vi "TLCamera Main.vi"() -> ()   [LabVIEW 2015]
uses:
  Status - Main.ctl
  Controls/Color Modes.ctl
  SubVIs/Parameters Get & Set/Get Parameters/Get CameraSensorType.vi
  Controls/Binning.ctl
  C:/code/Host/Installer/Scientific Camera Interfaces/LabVIEW/32_bit/Library_X86/Thorlabs.TSI.TLCameraInterfaces.dll
  code/Host/Installer/Scientific Camera Interfaces/LabVIEW/32_bit/Library_X86/Thorlabs.TSI.TLCameraInterfaces.dll
  Controls/Trigger Modes.ctl
  Controls/Taps.ctl
  SubVIs/Parameters Get & Set/Set Parameters/Set ExposureTime_us.vi
  SubVIs/Parameters Get & Set/Set Parameters/Set BlackLevel.vi
  SubVIs/Parameters Get & Set/Set Parameters/Set Gain.vi
  SubVIs/Parameters Get & Set/Get Parameters/Get ROIAndBin.vi
  SubVIs/Parameters Get & Set/Get Parameters/Get SensorHeight_pixels.vi
  SubVIs/Parameters Get & Set/Get Parameters/Get BinYRange.vi
  SubVIs/Parameters Get & Set/Get Parameters/Get BinXRange.vi
  SubVIs/Parameters Get & Set/Set Parameters/Set FramesPerTrigger_zeroForUnlimited.vi
  SubVIs/Parameters Get & Set/Set Parameters/Set DataRate.vi
  SubVIs/Parameters Get & Set/Set Parameters/Set ROIAndBin.vi
  SubVIs/Parameters Get & Set/Get Parameters/Get BlackLevelRange.vi
  SubVIs/Parameters Get & Set/Get Parameters/Get ExposureTimeRange_us.vi
  SubVIs/Parameters Get & Set/Get Parameters/Get GainRange.vi
  C:/code/Host/Installer/Scientific Camera Interfaces/LabVIEW/32_bit/Library_X86/Thorlabs.TSI.Demosaicker.dll
  code/Host/Installer/Scientific Camera Interfaces/LabVIEW/32_bit/Library_X86/Thorlabs.TSI.Demosaicker.dll
  C:/code/Host/Installer/Scientific Camera Interfaces/LabVIEW/32_bit/Library_X86/Thorlabs.TSI.ColorProcessor.dll
  code/Host/Installer/Scientific Camera Interfaces/LabVIEW/32_bit/Library_X86/Thorlabs.TSI.ColorProcessor.dll
  C:/code/Host/Installer/Scientific Camera Interfaces/LabVIEW/32_bit/Library_X86/Thorlabs.TSI.ColorInterfaces.dll
  code/Host/Installer/Scientific Camera Interfaces/LabVIEW/32_bit/Library_X86/Thorlabs.TSI.ColorInterfaces.dll
  SubVIs/Color/Color Processor References.ctl
  SubVIs/Parameters Get & Set/Get Parameters/Get BitDepth.vi
  Controls/Color Balance.ctl
  SubVIs/Parameters Get & Set/Set Parameters/Set Taps.vi
  SubVIs/Parameters Get & Set/Get Parameters/Get SensorWidth_pixels.vi
  Controls/Region of Interest.ctl
  Controls/Trigger Polarity.ctl
  Controls/Trigger Settings.ctl
  Controls/Data Rate.ctl
panel:
  out "event callback refnum":refnum<k27>
  out "Status":T1
  in  "Exit":bool
  out "Frame Number":u32
  out "Camera Image":picture
  in  "Camera Settings":T11={"Color Balance"={"Red Gain"=1.0, "Green Gain"=1.0, "Blue Gain"=1.0}, "Region of Interest"={"Origin - X"=0, "Origin - Y"=0, "Width"=1392, "Height"=1040}, "Binning"={"Bin - X"=1, "Bin - Y"=1}, "Frame Settings"={"Frames per Trigger\n(zero for unlimited)"=0}, "Data Rate"={"DataRate"=enum."ReadoutSpeed20MHz", "Taps"=enum."SingleTap"}, "Image Type"=enum."Standard RGB", "Trigger Settings"={"Trigger Mode"=enum."Software", "Trigger Polarity"=enum."ActiveHigh"}, "Exposure (ms)"=100.0, "Gain"=0, "Black Level"=48} {"Black Level" max=100; "Gain" max=1023; "Binning"."Bin - Y" min=1 max=16; "Binning"."Bin - X" min=1 max=16; "Color Balance"."Blue Gain" min=0 max=10 step=0.05 scale=0.0..10.0 scale format="%#_3g"; "Color Balance"."Green Gain" min=0 max=10 step=0.05 scale=0.0..10.0 scale format="%#_3g"; "Color Balance"."Red Gain" min=0 max=10 step=0.05 scale=0.0..10.0 scale format="%#_3g"}
  in  "Close Camera":bool
  in  "Open Camera":bool
  in  "Stop Camera":bool
  in  "Start Camera":bool
  in  "Refresh":bool
  in  "Camera Serial Numbers":u16(ring) items=["1234"]
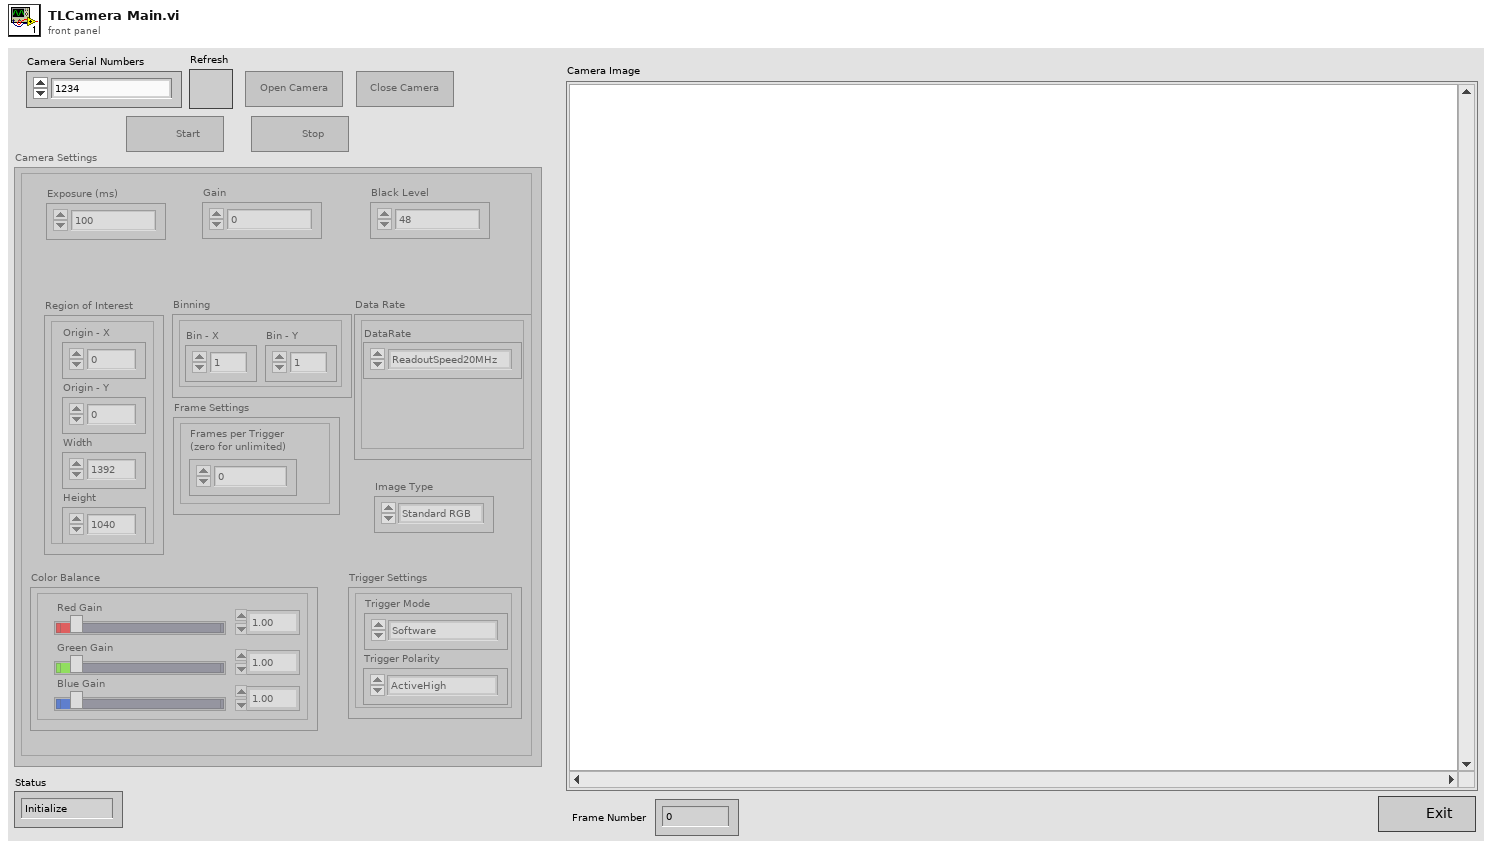
[diagram p1: front panel]
types:
  T1 = typedef "Status - Main.ctl" = enum16{"Initialize", "GUI", "Close"}
  T2 = typedef "Color Balance.ctl" = cluster{"Red Gain":sgl, "Green Gain":sgl, "Blue Gain":sgl}
  T3 = typedef "Region of Interest.ctl" = cluster{"Origin - X":u32, "Origin - Y":u32, "Width":u32, "Height":u32}
  T4 = typedef "Binning.ctl" = cluster{"Bin - X":u32, "Bin - Y":u32}
  T5 = typedef "Data Rate.ctl" = enum32{"ReadoutSpeed20MHz", "ReadoutSpeed40MHz", "FPS30", "FPS50"}
  T6 = typedef "Taps.ctl" = enum32{"SingleTap", "DualTap", "QuadTap"}
  T7 = typedef "Color Modes.ctl" = enum16{"Standard RGB", "Linear RGB", "Unprocessed"}
  T8 = typedef "Trigger Settings.ctl" = cluster{"Trigger Mode":T9, "Trigger Polarity":T10}
  T9 = typedef "Trigger Modes.ctl" = enum16{"Software", "Hardware Standard", "Bulb(PDX) Mode"}
  T10 = typedef "Trigger Polarity.ctl" = enum32{"ActiveHigh", "ActiveLow"}
  T11 = cluster{"Color Balance":T2, "Region of Interest":T3, "Binning":T4, "Frame Settings":cluster{"Frames per Trigger\n(zero for unlimited)":u32}, "Data Rate":cluster{"DataRate":T5, "Taps":T6}, "Image Type":T7, "Trigger Settings":T8, "Exposure (ms)":dbl, "Gain":u32, "Black Level":u32}
  T12 = typedef "Color Processor References.ctl" = cluster{"Demosaicker reference":refnum<k24>, "ColorProcessorSDK reference":refnum<k24>, "StandardRGBColorProcessor":refnum<k24>, "LinearRGBColorProcessor":refnum<k24>}
  T13 = enum8{"Enabled", "Disabled", "Disabled and Grayed Out"}
  T14 = cluster{"TLCamera reference out":refnum<k24>, "Frame Number":refnum<vi>, "Camera Image":refnum<vi>, "Value":T7, "Color Processor References":T12}
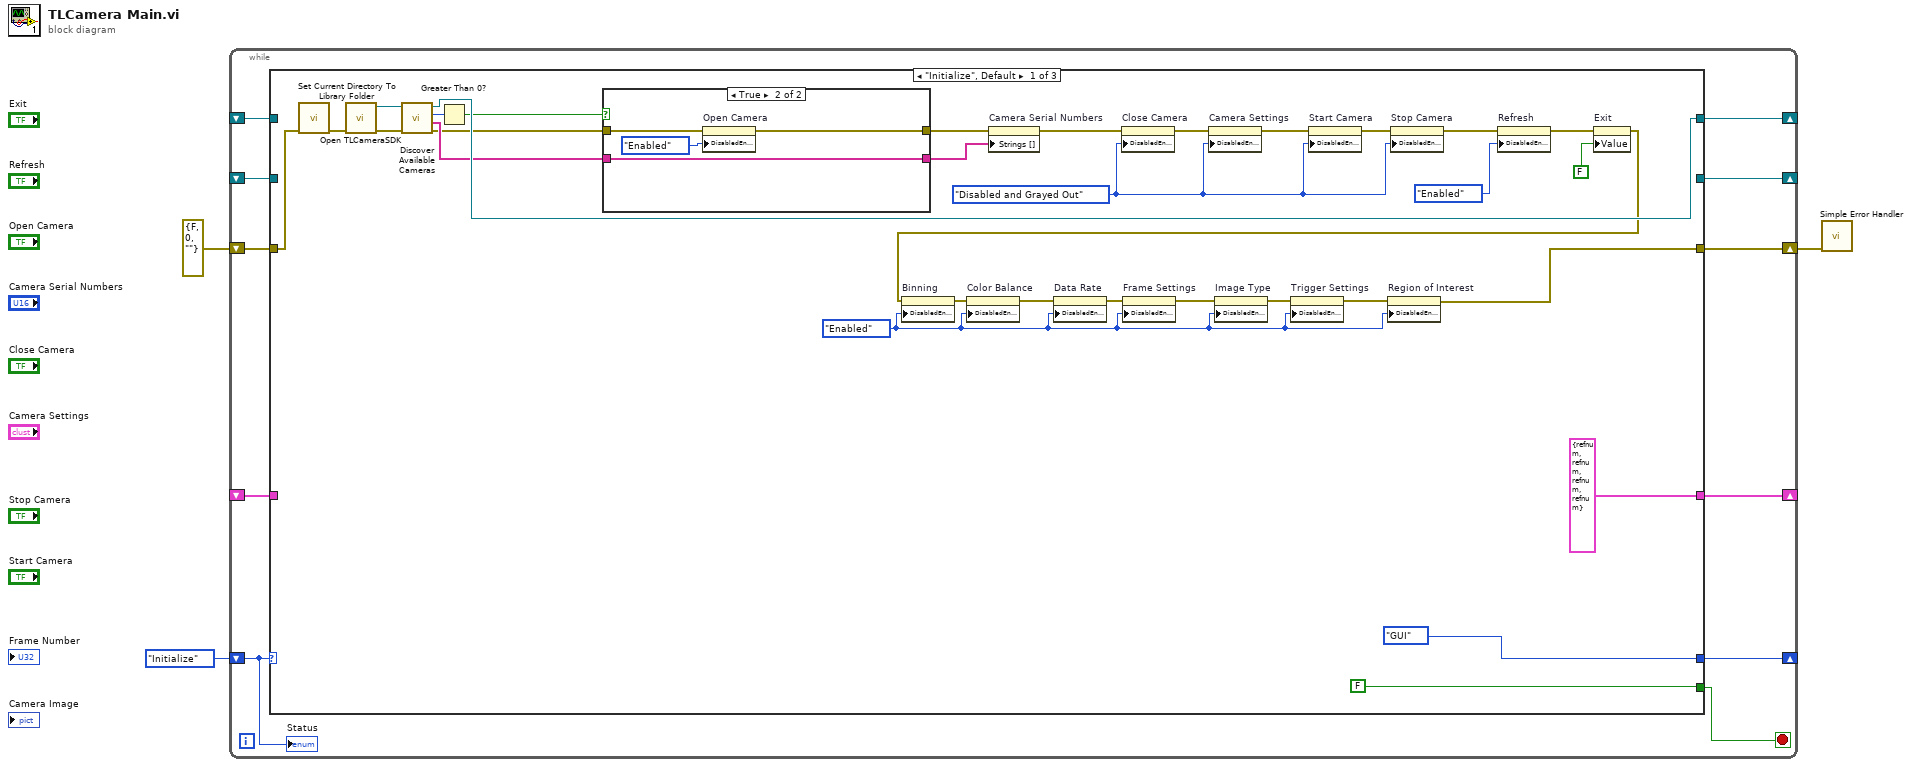
[diagram p0: block diagram]
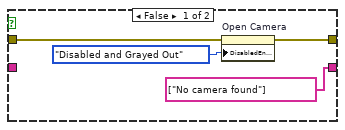
[diagram p2: hidden frame]
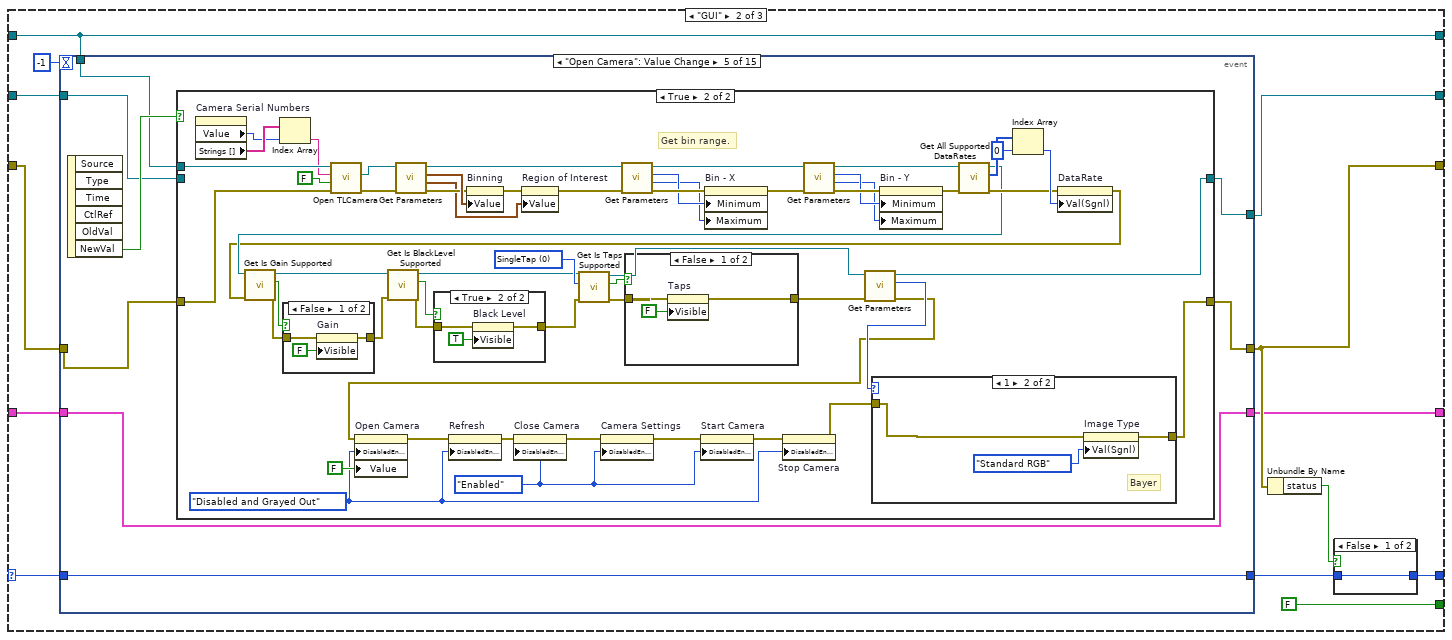
[diagram p3: hidden frame]
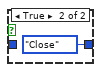
[diagram p4: hidden frame]
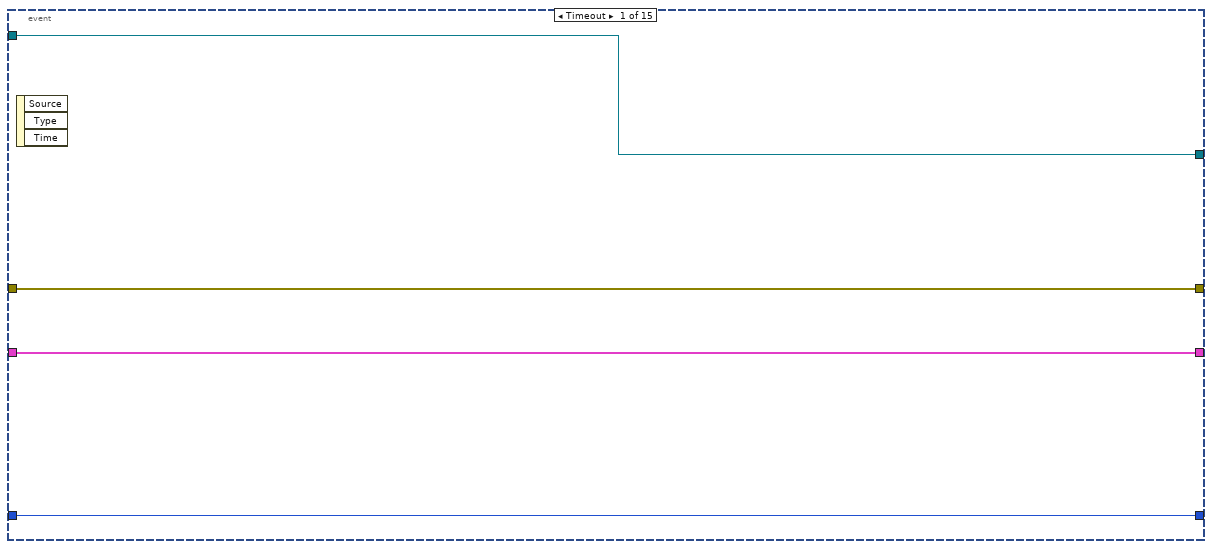
[diagram p5: hidden frame]
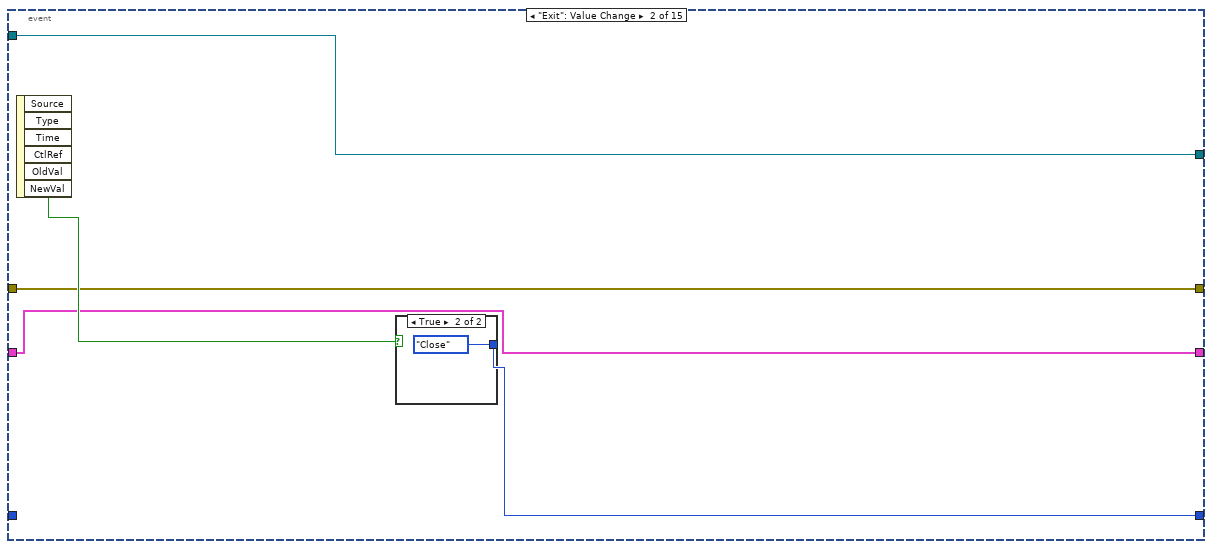
[diagram p6: hidden frame]
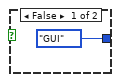
[diagram p7: hidden frame]
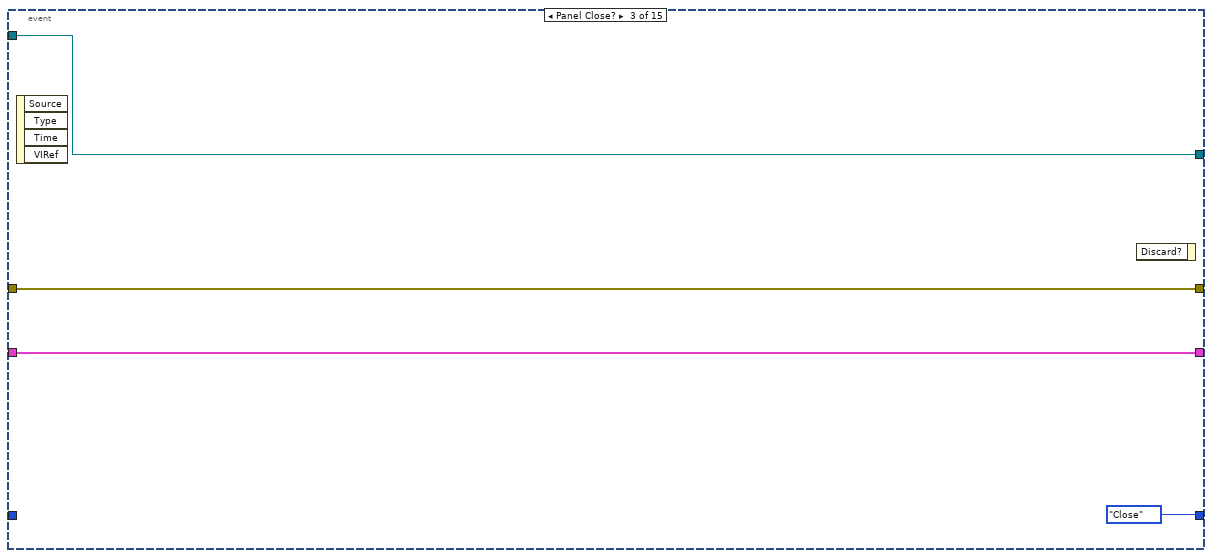
[diagram p8: hidden frame]
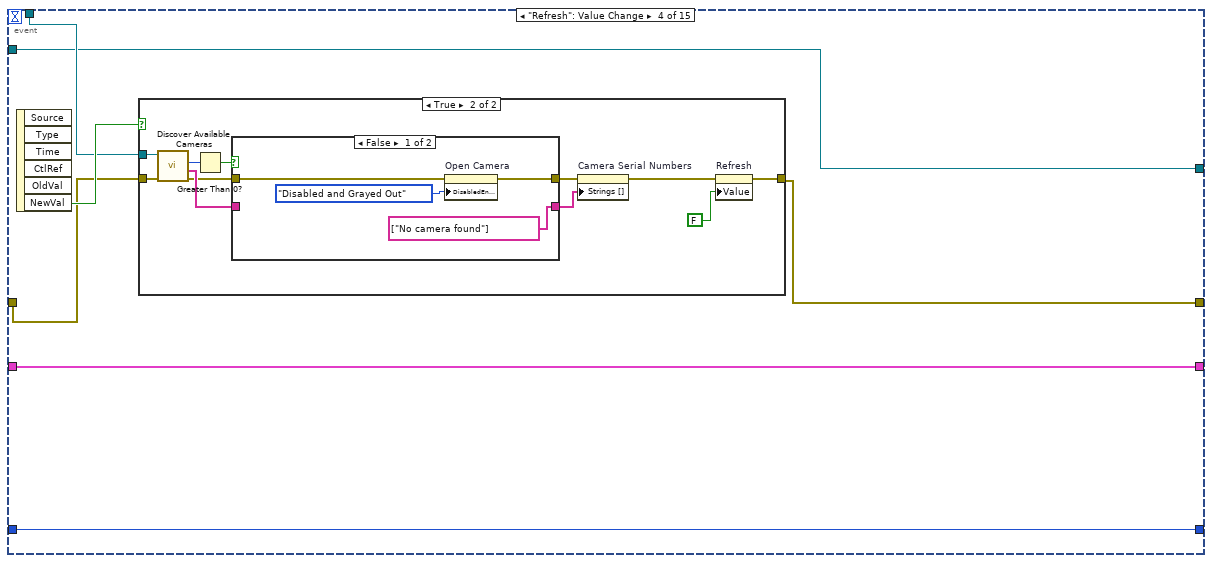
[diagram p9: hidden frame]
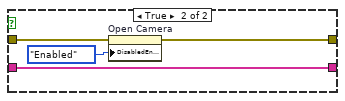
[diagram p11: hidden frame]
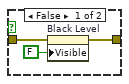
[diagram p13: hidden frame]
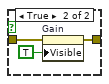
[diagram p14: hidden frame]
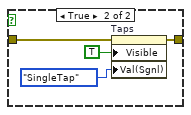
[diagram p15: hidden frame]
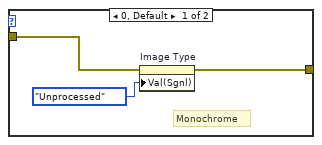
[diagram p16: hidden frame]
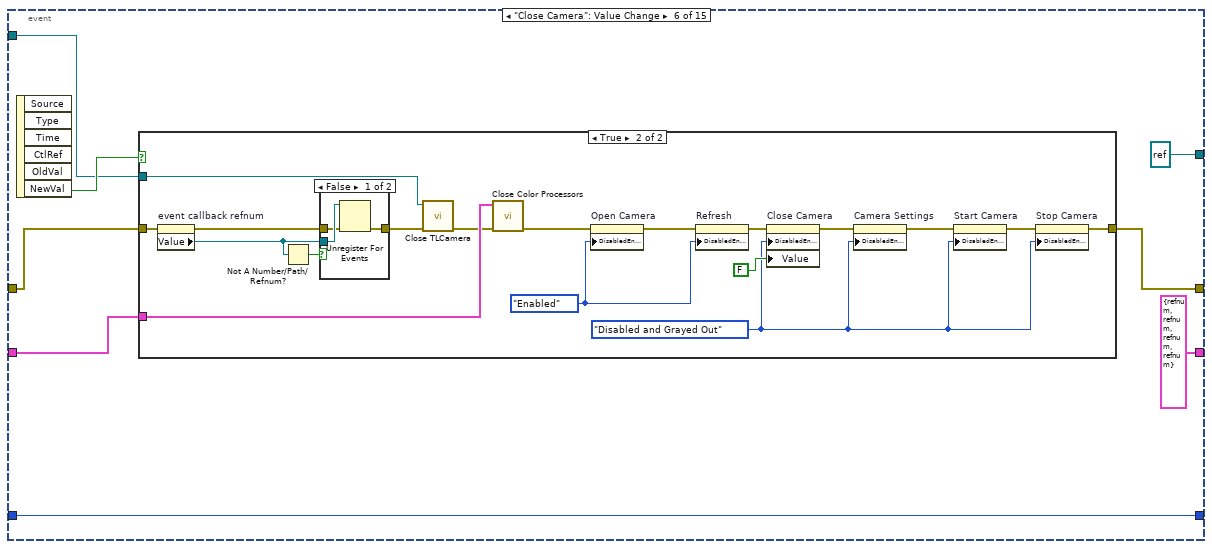
[diagram p17: hidden frame]
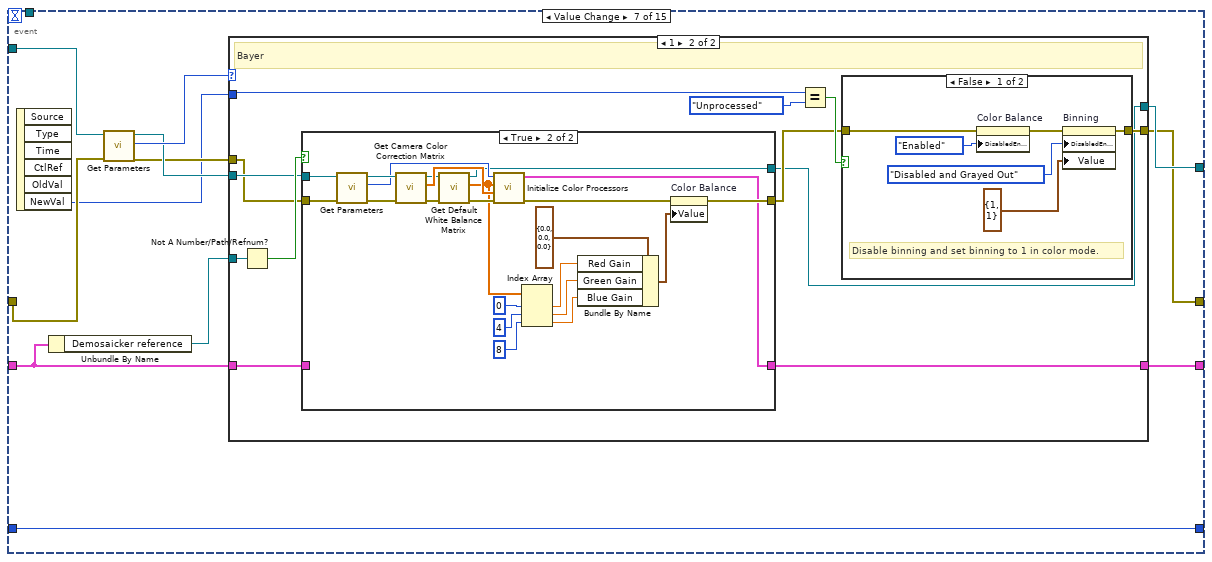
[diagram p20: hidden frame]
diagram:
  n1 = while {
    shift-right: [w7] -> _
    shift-left: Status_-_Main."Initialize" -> [w6]
    shift-right: [w14] -> _
    shift-left: _ -> [w13]
    shift-right: [w11] -> w1
    shift-left: errorcluster {"status"=FALSE, "code"=0, "source"=""} ("error in (no error)") -> [w12]
    shift-right: [w9] -> _
    shift-left: _ -> [w8]
    shift-right: [w4] -> _
    shift-left: _ -> [w5]
    stop <- w10 stop-if-true
    n2 = case shown="\"Initialize\", Default" w6 {
      selector: w6 -> [_ w65 w579]
      tunnel: [w45 w64 _] -> w14
      tunnel: w13 -> [_ w64 w581]
      tunnel: w12 -> [w17 w62 w562]
      tunnel: [w19 w61 w557] -> w11
      tunnel: [FALSE FALSE TRUE] -> w10
      tunnel: [Status_-_Main."GUI" w58 w579] -> w7
      tunnel: [_ w63 _] -> w9
      tunnel: w8 -> [_ w57 w576]
      tunnel: w5 -> [_ w56 w554]
      tunnel: [T12 {"Demosaicker reference"=refnum, "ColorProcessorSDK reference"=refnum, "StandardRGBColorProcessor"=refnum, "LinearRGBColorProcessor"=refnum} ("Color Processor References") w55 T12 {"Demosaicker reference"=refnum, "ColorProcessorSDK reference"=refnum, "StandardRGBColorProcessor"=refnum, "LinearRGBColorProcessor"=refnum} ("Color Processor References")] -> w4
      frame "Initialize", Default {
        w26 = T13."Enabled" ("Disabled")
        w35 = T13."Disabled and Grayed Out" ("Disabled")
        n3 = call "Set Current Directory To Library Folder.vi"("error in (no error)"=w17) -> ("error out"=w18:errorcluster)  [unwired: 10 in]
        n4 = call "Open TLCameraSDK.vi"("error in (no error)"=w18) -> ("error out"=w31:errorcluster, "TLCameraSDK ref out"=w30:refnum<k24>)  [unwired: 9 in]
        n5 = call "Discover Available Cameras.vi"("error in (no error)"=w31, "TLCameraSDK reference"=w30) -> ("error out"=w41:errorcluster, "Serial Numbers"=w43:string[], "Number of Cameras"=w46:i32, "TLCameraSDK reference out"=w45:refnum<k24>)  [unwired: 6 in]
        n6 = Greater Than 0?(x=w46) -> (x > 0?=w44:bool)
        n7 = case shown="True" w44 {
          tunnel: w43 -> [_ w54]
          tunnel: [string[] ["No camera found"] ("Serial Numbers") w54] -> w42
          tunnel: w41 -> [w48 w52]
          tunnel: [w47 w51] -> w40
          frame False {
            n8 = property on="Open Camera" class="Bool (strict)"(error in=w48, "DisabledEnum"=T13."Disabled and Grayed Out" ("Disabled")) -> (error out=w47:errorcluster)  [unwired: 1 in, 1 out]
          }
          frame True {
            n9 = property on="Open Camera" class="Bool (strict)"(error in=w52, "DisabledEnum"=T13."Enabled" ("Disabled")) -> (error out=w51:errorcluster)  [unwired: 1 in, 1 out]
          }
        }
        n10 = property on="Camera Serial Numbers" class="Ring (strict)"(error in=w40, "Strings []"=w42) -> (error out=w39:errorcluster)  [unwired: 1 in, 1 out]
        n11 = property on="Close Camera" class="Bool (strict)"(error in=w39, "DisabledEnum"=w35) -> (error out=w38:errorcluster)  [unwired: 1 in, 1 out]
        n12 = property on="Camera Settings" class="Clust (strict)"(error in=w38, "DisabledEnum"=w35) -> (error out=w37:errorcluster)  [unwired: 1 in, 1 out]
        n13 = property on="Start Camera" class="Bool (strict)"(error in=w37, "DisabledEnum"=w35) -> (error out=w36:errorcluster)  [unwired: 1 in, 1 out]
        n14 = property on="Stop Camera" class="Bool (strict)"(error in=w36, "DisabledEnum"=w35) -> (error out=w29:errorcluster)  [unwired: 1 in, 1 out]
        n15 = property on="Refresh" class="Bool (strict)"(error in=w29, "DisabledEnum"=T13."Enabled" ("Disabled")) -> (error out=w28:errorcluster)  [unwired: 1 in, 1 out]
        n16 = property on="Exit" class="Bool (strict)"(error in=w28, "Value"=FALSE ("Camera Running")) -> (error out=w25:errorcluster)  [unwired: 1 in, 1 out]
        n17 = property on="Binning" class="Clust (strict)"(error in=w25, "DisabledEnum"=w26) -> (error out=w24:errorcluster)  [unwired: 1 in, 1 out]
        n18 = property on="Color Balance" class="Clust (strict)"(error in=w24, "DisabledEnum"=w26) -> (error out=w23:errorcluster)  [unwired: 1 in, 1 out]
        n19 = property on="Data Rate" class="Clust (strict)"(error in=w23, "DisabledEnum"=w26) -> (error out=w16:errorcluster)  [unwired: 1 in, 1 out]
        n20 = property on="Frame Settings" class="Clust (strict)"(error in=w16, "DisabledEnum"=w26) -> (error out=w22:errorcluster)  [unwired: 1 in, 1 out]
        n21 = property on="Image Type" class="Enum (strict)"(error in=w22, "DisabledEnum"=w26) -> (error out=w21:errorcluster)  [unwired: 1 in, 1 out]
        n22 = property on="Trigger Settings" class="Clust (strict)"(error in=w21, "DisabledEnum"=w26) -> (error out=w20:errorcluster)  [unwired: 1 in, 1 out]
        n23 = property on="Region of Interest" class="Clust (strict)"(error in=w20, "DisabledEnum"=w26) -> (error out=w19:errorcluster)  [unwired: 1 in, 1 out]
      }
      frame "GUI" {
        n24 = event shown="[4] \"Open Camera\": Value Change" {
          selector: _ -> [_ _ _ _ _ _ _ _ _ _ _ _ _ _ _]
          dyn-events: _ -> [_ _ _ _ _ _ _ _ _ _ _ _ _ _ _]
          timeout: -1 -> [_ _ _ _ _ _ _ _ _ _ _ _ _ _ _]
          tunnel: [w73 w77 Status_-_Main."Close" w87 w117 w206 w245 w316 w328 w347 w364 w395 w422 w487 w525] -> w59
          tunnel: w65 -> [w73 _ _ w87 w117 w206 w245 w316 w328 w347 w364 w395 w422 w487 w525]
          tunnel: w64 -> [_ _ _ w90 w118 _ _ _ _ _ _ _ _ _ _]
          tunnel: w62 -> [w72 w76 w83 w89 w116 w209 w244 w315 w331 w343 w366 w383 w420 w426 w528]
          tunnel: [w71 w75 w82 w86 w115 refnum<k24> refnum ("TLCamera reference") w239 w307 w319 w336 w356 w378 w423 w474 w527] -> w63
          tunnel: [w72 w76 w83 w88 w114 w208 w238 w308 w318 w335 w357 w379 w424 w471 w526] -> w61
          tunnel: w57 -> [w71 w75 w82 w86 w113 w205 w237 w306 w327 w342 w367 w378 w421 w472 w524]
          tunnel: w56 -> [w70 w74 w81 w85 w112 w203 w234 w304 w317 w333 w355 w377 w418 w437 w522]
          tunnel: [w70 w74 w81 w85 w112 T12 {"Demosaicker reference"=refnum, "ColorProcessorSDK reference"=refnum, "StandardRGBColorProcessor"=refnum, "LinearRGBColorProcessor"=refnum} ("Color Processor References") w235 w304 w317 w333 w355 w377 w418 w437 w522] -> w55
          event Timeout {
            n25 = event-data() -> ()  [unwired: 1 in, 3 out]
          }
          event "Exit": Value Change {
            n26 = event-data() -> ("NewVal"=w78:bool)  [unwired: 1 in, 5 out]
            n27 = case shown="True" w78 {
              tunnel: [Status_-_Main."GUI" Status_-_Main."Close"] -> w77
              frame False {
              }
              frame True {
              }
            }
          }
          event Panel Close? {
            n28 = event-data() -> ()  [unwired: 1 in, 4 out]
            n29 = event-data() -> ()  [unwired: 2 in, 1 out]
          }
          event "Refresh": Value Change {
            n30 = event-data() -> ("NewVal"=w91:bool)  [unwired: 1 in, 5 out]
            n31 = case shown="True" w91 {
              tunnel: w90 -> [_ w103]
              tunnel: w89 -> [w92 w102]
              tunnel: [w92 w93] -> w88
              frame False {
              }
              frame True {
                n32 = call "Discover Available Cameras.vi"("error in (no error)"=w102, "TLCameraSDK reference"=w103) -> ("error out"=w99:errorcluster, "Serial Numbers"=w100:string[], "Number of Cameras"=w101:i32)  [unwired: 6 in, 1 out]
                n33 = Greater Than 0?(x=w101) -> (x > 0?=w96:bool)
                n34 = case shown="False" w96 {
                  tunnel: w100 -> [_ w111]
                  tunnel: [string[] ["No camera found"] ("Serial Numbers") w111] -> w98
                  tunnel: w99 -> [w105 w109]
                  tunnel: [w104 w108] -> w97
                  frame False {
                    n35 = property on="Open Camera" class="Bool (strict)"(error in=w105, "DisabledEnum"=T13."Disabled and Grayed Out" ("Disabled")) -> (error out=w104:errorcluster)  [unwired: 1 in, 1 out]
                  }
                  frame True {
                    n36 = property on="Open Camera" class="Bool (strict)"(error in=w109, "DisabledEnum"=T13."Enabled" ("Disabled")) -> (error out=w108:errorcluster)  [unwired: 1 in, 1 out]
                  }
                }
                n37 = property on="Camera Serial Numbers" class="Ring (strict)"(error in=w97, "Strings []"=w98) -> (error out=w94:errorcluster)  [unwired: 1 in, 1 out]
                n38 = property on="Refresh" class="Bool (strict)"(error in=w94, "Value"=FALSE ("Refresh")) -> (error out=w93:errorcluster)  [unwired: 1 in, 1 out]
              }
            }
          }
          event "Open Camera": Value Change {
            n39 = event-data() -> ("NewVal"=w119:bool)  [unwired: 1 in, 5 out]
            n40 = case shown="True" w119 {
              tunnel: w118 -> [_ w177]
              tunnel: w116 -> [w120 w145]
              tunnel: [w121 w123] -> w115
              tunnel: w113 -> [w121 _]
              tunnel: [w120 w146] -> w114
              frame False {
              }
              frame True {
                w144 = 0 items=["SingleTap", "DualTap", "QuadTap"] ("Taps")
                w164 = T13."Enabled" ("Disabled")
                w165 = T13."Disabled and Grayed Out" ("Disabled")
                # "Get bin range."
                n41 = property on="Camera Serial Numbers" class="Ring (strict)"() -> ("Value"=w175:u16, "Strings []"=w176:string[])  [unwired: 2 in, 2 out]
                n42 = Index Array(array=w176, index=w175) -> (element=w174:string)
                n43 = call "Open TLCamera.vi"("error in (no error)"=w145, "isDiagnosticsMessagesEnabled"=FALSE, "Camera serial number"=w174, "TLCameraSDK reference"=w177) -> ("error out"=w162:errorcluster, "TLCamera reference out"=w161:refnum<k24>)  [unwired: 5 in, 1 out]
                n44 = call-poly "Get Parameters.vi"("error in (no error)"=w162, "TLCamera reference in"=w161) -> ("error out"=w159:errorcluster, "Region of Interest"=w158:T3, "Binning"=w160:T4, "TLCamera reference out"=w147:refnum<k24>)  [unwired: 6 in]
                n45 = property on="Binning" class="Clust (strict)"(error in=w159, "Value"=w160) -> (error out=w157:errorcluster)  [unwired: 1 in, 1 out]
                n46 = property on="Region of Interest" class="Clust (strict)"(error in=w157, "Value"=w158) -> (error out=w148:errorcluster)  [unwired: 1 in, 1 out]
                n47 = call-poly "Get Parameters.vi"("error in (no error)"=w148, "TLCamera reference in"=w147) -> ("error out"=w156:errorcluster, "Maximum"=w154:u32, "Minimum"=w155:u32, "TLCamera reference out"=w152:refnum<k24>)  [unwired: 6 in]
                n48 = property on="Bin - X" class="DigNum (strict)"(error in=w156, "Minimum"=w155, "Maximum"=w154) -> (error out=w153:errorcluster)  [unwired: 1 in, 1 out]
                n49 = call-poly "Get Parameters.vi"("error in (no error)"=w153, "TLCamera reference in"=w152) -> ("error out"=w151:errorcluster, "Maximum"=w149:u32, "Minimum"=w150:u32, "TLCamera reference out"=w143:refnum<k24>)  [unwired: 6 in]
                n50 = property on="Bin - Y" class="DigNum (strict)"(error in=w151, "Minimum"=w150, "Maximum"=w149) -> (error out=w142:errorcluster)  [unwired: 1 in, 1 out]
                n51 = call "Get All Supported DataRates.vi"("error in (no error)"=w142, "TLCamera reference"=w143) -> ("error out"=w138:errorcluster, "Supported DataRates"=w141:i32[], "TLCamera reference out"=w133:refnum<k24>)  [unwired: 7 in]
                n52 = Index Array(array=w141, index=0) -> (element=w139:i32)
                n53 = property on="DataRate" class="Enum (strict)"(error in=w138, "Val(Sgnl)"=w139) -> (error out=w132:errorcluster)  [unwired: 1 in, 1 out]
                n54 = call "Get Is Gain Supported.vi"("error in (no error)"=w132, "TLCamera reference in"=w133) -> ("error out"=w130:errorcluster, "Is Gain Supported?"=w131:bool, "TLCamera reference out"=w128:refnum<k24>)  [unwired: 7 in]
                n55 = case shown="False" w131 {
                  tunnel: w130 -> [w185 w189]
                  tunnel: [w184 w187] -> w129
                  frame False {
                    n56 = property on="Gain" class="DigNum (strict)"(error in=w185, "Visible"=FALSE) -> (error out=w184:errorcluster)  [unwired: 1 in, 1 out]
                  }
                  frame True {
                    n57 = property on="Gain" class="DigNum (strict)"(error in=w189, "Visible"=TRUE) -> (error out=w187:errorcluster)  [unwired: 1 in, 1 out]
                  }
                }
                n58 = call "Get Is BlackLevel Supported.vi"("error in (no error)"=w129, "TLCamera reference in"=w128) -> ("error out"=w126:errorcluster, "Is BlackLevel Supported?"=w127:bool, "TLCamera reference out"=w124:refnum<k24>)  [unwired: 7 in]
                n59 = case shown="True" w127 {
                  tunnel: w126 -> [w179 w183]
                  tunnel: [w178 w181] -> w125
                  frame False {
                    n60 = property on="Black Level" class="DigNum (strict)"(error in=w179, "Visible"=FALSE) -> (error out=w178:errorcluster)  [unwired: 1 in, 1 out]
                  }
                  frame True {
                    n61 = property on="Black Level" class="DigNum (strict)"(error in=w183, "Visible"=TRUE) -> (error out=w181:errorcluster)  [unwired: 1 in, 1 out]
                  }
                }
                n62 = call "Get Is Taps Supported.vi"("error in (no error)"=w125, "Taps"=w144, "TLCamera reference"=w124) -> ("error out"=w136:errorcluster, "Is Taps Supported"=w137:bool, "TLCamera reference out"=w135:refnum<k24>)  [unwired: 6 in]
                n63 = case shown="False" w137 {
                  tunnel: w136 -> [w191 w196]
                  tunnel: [w190 w195] -> w134
                  frame False {
                    n64 = property on="Taps" class="Enum (strict)"(error in=w191, "Visible"=FALSE) -> (error out=w190:errorcluster)  [unwired: 1 in, 1 out]
                  }
                  frame True {
                    n65 = property on="Taps" class="Enum (strict)"(error in=w196, "Visible"=TRUE, "Val(Sgnl)"=Taps."SingleTap" ("Value (Signaling)")) -> (error out=w195:errorcluster)  [unwired: 1 in, 1 out]
                  }
                }
                n66 = call-poly "Get Parameters.vi"("error in (no error)"=w134, "TLCamera reference in"=w135) -> ("error out"=w122:errorcluster, "CameraSensorType"=w163:i32, "TLCamera reference out"=w123:refnum<k24>)  [unwired: 7 in]
                n67 = property on="Open Camera" class="Bool (strict)"(error in=w122, "DisabledEnum"=w165, "Value"=FALSE ("Open Camera")) -> (error out=w170:errorcluster)  [unwired: 1 in, 1 out]
                n68 = property on="Refresh" class="Bool (strict)"(error in=w170, "DisabledEnum"=w165) -> (error out=w169:errorcluster)  [unwired: 1 in, 1 out]
                n69 = property on="Close Camera" class="Bool (strict)"(error in=w169, "DisabledEnum"=w164) -> (error out=w171:errorcluster)  [unwired: 1 in, 1 out]
                n70 = property on="Camera Settings" class="Clust (strict)"(error in=w171, "DisabledEnum"=w164) -> (error out=w168:errorcluster)  [unwired: 1 in, 1 out]
                n71 = property on="Start Camera" class="Bool (strict)"(error in=w168, "DisabledEnum"=w164) -> (error out=w167:errorcluster)  [unwired: 1 in, 1 out]
                n72 = property on="Stop Camera" class="Bool (strict)"(error in=w167, "DisabledEnum"=w165) -> (error out=w166:errorcluster)  [unwired: 1 in, 1 out]
                n73 = case shown="1" w163 {
                  tunnel: w166 -> [w197 w200]
                  tunnel: [w199 w202] -> w146
                  frame 0, Default {
                    # "Monochrome"
                    n74 = property on="Image Type" class="Enum (strict)"(error in=w197, "Val(Sgnl)"=Color_Modes."Unprocessed" ("Value")) -> (error out=w199:errorcluster)  [unwired: 1 in, 1 out]
                  }
                  frame 1 {
                    # "Bayer"
                    n75 = property on="Image Type" class="Enum (strict)"(error in=w200, "Val(Sgnl)"=Color_Modes."Standard RGB" ("Value")) -> (error out=w202:errorcluster)  [unwired: 1 in, 1 out]
                  }
                }
              }
            }
          }
          event "Close Camera": Value Change {
            n76 = event-data() -> ("NewVal"=w210:bool)  [unwired: 1 in, 5 out]
            n77 = case shown="True" w210 {
              tunnel: w205 -> [_ w229]
              tunnel: w209 -> [w211 w218]
              tunnel: [w211 w222] -> w208
              tunnel: w203 -> [_ w214]
              frame False {
              }
              frame True {
                w215 = T13."Disabled and Grayed Out" ("Disabled")
                w223 = T13."Enabled" ("Disabled")
                n78 = property on="event callback refnum" class="Ref (strict)"(error in=w218) -> (error out=w219:errorcluster, "Value"=w220:refnum<k27>)  [unwired: 1 in, 1 out]
                n79 = Not A Number/Path/Refnum?(number/path/refnum=w220) -> (NaN/Path/Refnum?=w221:bool)
                n80 = case shown="False" w221 {
                  tunnel: w220 -> [w232 _]
                  tunnel: w219 -> [w231 w233]
                  tunnel: [w230 w233] -> w217
                  frame False {
                    n81 = Unregister For Events(event registration refnum=w232, error in=w231) -> (error out=w230:errorcluster)
                  }
                  frame True {
                  }
                }
                n82 = call "Close TLCamera.vi"("error in (no error)"=w217, "TLCamera reference"=w229) -> ("error out"=w213:errorcluster)  [unwired: 9 in]
                n83 = call "Close Color Processors.vi"("error in (no error)"=w213, "Color Processor References"=w214) -> ("error out"=w212:errorcluster)  [unwired: 9 in]
                n84 = property on="Open Camera" class="Bool (strict)"(error in=w212, "DisabledEnum"=w223) -> (error out=w225:errorcluster)  [unwired: 1 in, 1 out]
                n85 = property on="Refresh" class="Bool (strict)"(error in=w225, "DisabledEnum"=w223) -> (error out=w224:errorcluster)  [unwired: 1 in, 1 out]
                n86 = property on="Close Camera" class="Bool (strict)"(error in=w224, "DisabledEnum"=w215, "Value"=FALSE ("Close Camera")) -> (error out=w228:errorcluster)  [unwired: 1 in, 1 out]
                n87 = property on="Camera Settings" class="Clust (strict)"(error in=w228, "DisabledEnum"=w215) -> (error out=w216:errorcluster)  [unwired: 1 in, 1 out]
                n88 = property on="Start Camera" class="Bool (strict)"(error in=w216, "DisabledEnum"=w215) -> (error out=w226:errorcluster)  [unwired: 1 in, 1 out]
                n89 = property on="Stop Camera" class="Bool (strict)"(error in=w226, "DisabledEnum"=w215) -> (error out=w222:errorcluster)  [unwired: 1 in, 1 out]
              }
            }
          }
          event Value Change {
            n90 = event-data() -> ("NewVal"=w240:T7)  [unwired: 1 in, 5 out]
            n91 = Unbundle By Name(w234) -> ("Demosaicker reference"=w236:refnum<k24>)
            n92 = call-poly "Get Parameters.vi"("error in (no error)"=w244, "TLCamera reference in"=w237) -> ("error out"=w241:errorcluster, "CameraSensorType"=w243:i32, "TLCamera reference out"=w242:refnum<k24>)  [unwired: 7 in]
            n93 = case shown="1" w243 {
              tunnel: w242 -> [w248 w261]
              tunnel: w241 -> [w251 w260]
              tunnel: w240 -> [_ w264]
              tunnel: [w248 w258] -> w239
              tunnel: [w252 w265] -> w238
              tunnel: w236 -> [_ w263]
              tunnel: [w246 w256] -> w235
              tunnel: w234 -> [w246 w257]
              frame 0, Default {
                # "Monochrome"
                n94 = property on="Image Type" class="Enum (strict)"(error in=w251, "Value"=Color_Modes."Unprocessed") -> (error out=w249:errorcluster)  [unwired: 1 in, 1 out]
                n95 = property on="Binning" class="Clust (strict)"(error in=w249, "DisabledEnum"=T13."Enabled" ("Disabled"), "Value"=T4 {"Bin - X"=1, "Bin - Y"=1}) -> (error out=w253:errorcluster)  [unwired: 1 in, 1 out]
                n96 = property on="Color Balance" class="Clust (strict)"(error in=w253, "DisabledEnum"=T13."Disabled and Grayed Out" ("Disabled")) -> (error out=w252:errorcluster)  [unwired: 1 in, 1 out]
              }
              frame 1 {
                # "Bayer"
                n97 = Not A Number/Path/Refnum?(number/path/refnum=w263) -> (NaN/Path/Refnum?=w262:bool)
                n98 = case shown="True" w262 {
                  tunnel: w261 -> [w269 w288]
                  tunnel: w260 -> [w270 w289]
                  tunnel: [w270 w273] -> w259
                  tunnel: [w269 w272] -> w258
                  tunnel: w257 -> [w268 _]
                  tunnel: [w268 w271] -> w256
                  frame False {
                  }
                  frame True {
                    n99 = call-poly "Get Parameters.vi"("error in (no error)"=w289, "TLCamera reference in"=w288) -> ("error out"=w286:errorcluster, "BitDepth"=w285:u32, "TLCamera reference out"=w287:refnum<k24>)  [unwired: 7 in]
                    n100 = call "Get Camera Color Correction Matrix.vi"("error in (no error)"=w286, "TLCamera reference"=w287) -> ("error out"=w291:errorcluster, "Camera Color Correction Matrix"=w292:sgl[], "TLCamera reference out"=w290:refnum<k24>)  [unwired: 7 in]
                    n101 = call "Get Default White Balance Matrix.vi"("error in (no error)"=w291, "TLCamera reference"=w290) -> ("error out"=w284:errorcluster, "Default White Balance Matrix"=w283:sgl[], "TLCamera reference out"=w272:refnum<k24>)  [unwired: 7 in]
                    n102 = call "Initialize Color Processors.vi"("error in (no error)"=w284, "Camera Color Correction Matrix"=w292, "White Balance Matrix"=w283, "BitDepth"=w285) -> ("error out"=w274:errorcluster, "Color Processor References"=w271:T12)  [unwired: 6 in]
                    n103 = Index Array(array=w283, index #1=0 ("index"), index #2=4 ("index"), index #3=8 ("index")) -> (element #1=w277:sgl, element #2=w276:sgl, element #3=w275:sgl)
                    n104 = Bundle By Name(cluster=T2 {"Red Gain"=0.0, "Green Gain"=0.0, "Blue Gain"=0.0} ("Value"), "Red Gain"=w277, "Green Gain"=w276, "Blue Gain"=w275) -> (w279:T2)
                    n105 = property on="Color Balance" class="Clust (strict)"(error in=w274, "Value"=w279) -> (error out=w273:errorcluster)  [unwired: 1 in, 1 out]
                  }
                }
                n106 = Equal?(x=w264, y=Color_Modes."Unprocessed") -> (x = y?=w266:bool)
                n107 = case shown="False" w266 {
                  tunnel: w259 -> [w293 w299]
                  tunnel: [w294 w300] -> w265
                  frame False {
                    # "Disable binning and set binning to 1 in color mode."
                    n108 = property on="Color Balance" class="Clust (strict)"(error in=w293, "DisabledEnum"=T13."Enabled" ("Disabled")) -> (error out=w298:errorcluster)  [unwired: 1 in, 1 out]
                    n109 = property on="Binning" class="Clust (strict)"(error in=w298, "DisabledEnum"=T13."Disabled and Grayed Out" ("Disabled"), "Value"=T4 {"Bin - X"=1, "Bin - Y"=1} ("Value (Signaling)")) -> (error out=w294:errorcluster)  [unwired: 1 in, 1 out]
                  }
                  frame True {
                    # "Enable binning and disable color balance"
                    n110 = property on="Binning" class="Clust (strict)"(error in=w299, "DisabledEnum"=T13."Enabled" ("Disabled")) -> (error out=w303:errorcluster)  [unwired: 1 in, 1 out]
                    n111 = property on="Color Balance" class="Clust (strict)"(error in=w303, "DisabledEnum"=T13."Disabled and Grayed Out" ("Disabled")) -> (error out=w300:errorcluster)  [unwired: 1 in, 1 out]
                  }
                }
              }
            }
          }
          event Value Change {
            n112 = event-data() -> ("NewVal"=w305:T3)  [unwired: 1 in, 5 out]
            n113 = call-poly "Get Parameters.vi"("error in (no error)"=w315, "TLCamera reference in"=w306) -> ("error out"=w313:errorcluster, "SensorHeight_pixels"=w311:u32, "TLCamera reference out"=w314:refnum<k24>)  [unwired: 7 in]
            n114 = call-poly "Get Parameters.vi"("error in (no error)"=w313, "TLCamera reference in"=w314) -> ("error out"=w309:errorcluster, "SensorWidth_pixels"=w312:u32, "TLCamera reference out"=w307:refnum<k24>)  [unwired: 7 in]
            n115 = call "Validate ROI.vi"("ROI in"=w305, "SensorHeight_pixels"=w311, "SensorWidth_pixels"=w312) -> ("ROI out"=w310:T3)  [unwired: 8 in]
            n116 = property on="Region of Interest" class="Clust (strict)"(error in=w309, "Value"=w310) -> (error out=w308:errorcluster)  [unwired: 1 in, 1 out]
          }
          event "Camera Settings.Exposure (ms)": Value Change {
            n117 = event-data() -> ("NewVal"=w326:dbl)  [unwired: 1 in, 5 out]
            n118 = call-poly "Get Parameters.vi"("error in (no error)"=w331, "TLCamera reference in"=w327) -> ("error out"=w323:errorcluster, "Maximum"=w329:u32, "TLCamera reference out"=w322:refnum<k24>)  [unwired: 6 in, 1 out]
            n119 = Multiply(x=1000.0, y=w326) -> (x*y=w330:dbl)
            n120 = Max & Min(x=w329, y=w330) -> (min(x,y)=w320:dbl)  [unwired: 1 out]
            n121 = Divide(x=w320, y=1000.0) -> (x/y=w324:dbl)
            n122 = property on="Exposure (ms)" class="DigNum (strict)"(error in=w323, "Value"=w324) -> (error out=w321:errorcluster)  [unwired: 1 in, 1 out]
            n123 = call-poly "Set Parameters.vi"("error in (no error)"=w321, "ExposureTime_us"=w320, "TLCamera reference in"=w322) -> ("error out"=w318:errorcluster, "TLCamera reference out"=w319:refnum<k24>)  [unwired: 7 in]
          }
          event "Camera Settings.Gain": Value Change {
            n124 = event-data() -> ("NewVal"=w344:u32)  [unwired: 1 in, 5 out]
            n125 = call-poly "Get Parameters.vi"("error in (no error)"=w343, "TLCamera reference in"=w342) -> ("error out"=w345:errorcluster, "Maximum"=w346:u32, "TLCamera reference out"=w341:refnum<k24>)  [unwired: 6 in, 1 out]
            n126 = Max & Min(x=w346, y=w344) -> (min(x,y)=w334:u32)  [unwired: 1 out]
            n127 = property on="Gain" class="DigNum (strict)"(error in=w345, "Value"=w334) -> (error out=w340:errorcluster)  [unwired: 1 in, 1 out]
            n128 = call "Get Is Gain Supported.vi"("error in (no error)"=w340, "TLCamera reference in"=w341) -> ("error out"=w337:errorcluster, "Is Gain Supported?"=w339:bool, "TLCamera reference out"=w338:refnum<k24>)  [unwired: 7 in]
            n129 = case shown="True" w339 {
              tunnel: w338 -> [w349 w354]
              tunnel: w337 -> [w348 w353]
              tunnel: [w349 w352] -> w336
              tunnel: [w348 w351] -> w335
              tunnel: w334 -> [_ w350]
              frame False {
              }
              frame True {
                n130 = call-poly "Set Parameters.vi"("error in (no error)"=w353, "Gain"=w350, "TLCamera reference in"=w354) -> ("error out"=w351:errorcluster, "TLCamera reference out"=w352:refnum<k24>)  [unwired: 7 in]
              }
            }
          }
          event "Camera Settings.Black Level": Value Change {
            n131 = event-data() -> ("NewVal"=w365:u32)  [unwired: 1 in, 5 out]
            n132 = call-poly "Get Parameters.vi"("error in (no error)"=w366, "TLCamera reference in"=w367) -> ("error out"=w368:errorcluster, "Maximum"=w369:u32, "TLCamera reference out"=w363:refnum<k24>)  [unwired: 6 in, 1 out]
            n133 = Max & Min(x=w369, y=w365) -> (min(x,y)=w358:u32)  [unwired: 1 out]
            n134 = property on="Black Level" class="DigNum (strict)"(error in=w368, "Value"=w358) -> (error out=w362:errorcluster)  [unwired: 1 in, 1 out]
            n135 = call "Get Is BlackLevel Supported.vi"("error in (no error)"=w362, "TLCamera reference in"=w363) -> ("error out"=w359:errorcluster, "Is BlackLevel Supported?"=w361:bool, "TLCamera reference out"=w360:refnum<k24>)  [unwired: 7 in]
            n136 = case shown="False" w361 {
              tunnel: w360 -> [w371 w376]
              tunnel: w359 -> [w370 w375]
              tunnel: w358 -> [_ w374]
              tunnel: [w370 w373] -> w357
              tunnel: [w371 w372] -> w356
              frame False {
              }
              frame True {
                n137 = call-poly "Set Parameters.vi"("error in (no error)"=w375, "BlackLevel"=w374, "TLCamera reference in"=w376) -> ("error out"=w373:errorcluster, "TLCamera reference out"=w372:refnum<k24>)  [unwired: 7 in]
              }
            }
          }
          event "Camera Settings.Data Rate": Value Change {
            n138 = event-data() -> ()  [unwired: 1 in, 6 out]
            n139 = property on="DataRate" class="Enum (strict)"(error in=w383) -> (error out=w384:errorcluster, "NumItems"=w394:u32, "Value"=w392:T5)  [unwired: 1 in, 1 out]
            n140 = property on="Taps" class="Enum (strict)"(error in=w383) -> (error out=w382:errorcluster, "NumItems"=w389:u32, "Value"=w387:T6)  [unwired: 1 in, 1 out]
            n141 = Initialize Array(w392) -> (w393:T5[])  [unwired: 1 in]
            n142 = Initialize Array(w387) -> (w388:T6[])  [unwired: 1 in]
            n143 = for {
              N: w394 -> [_]
              tunnel: w378 -> [w413]
              shift-right: [w409] -> w391
              shift-left: w393 -> [w410]
              shift-right: [w407] -> w390
              shift-left: w384 -> [w412]
              i -> [w408]
              n144 = call "Get Is DataRate Supported.vi"("error in (no error)"=w412, "Data Rate"=w408, "TLCamera reference"=w413) -> ("error out"=w407:errorcluster, "Is DataRate Supported"=w411:bool)  [unwired: 6 in, 1 out]
              n145 = case shown="False" w411 {
                tunnel: w410 -> [w416 w417]
                tunnel: [w414 w417] -> w409
                tunnel: w408 -> [w415 _]
                frame False {
                  n146 = Build Array (concatenate)(w416, w415) -> (w414:u32[])
                }
                frame True {
                }
              }
            }
            n147 = for {
              N: w389 -> [_]
              tunnel: w378 -> [w402]
              shift-right: [w398] -> w386
              shift-left: w388 -> [w399]
              shift-right: [w396] -> w385
              shift-left: w382 -> [w401]
              i -> [w397]
              n148 = call "Get Is Taps Supported.vi"("error in (no error)"=w401, "Taps"=w397, "TLCamera reference"=w402) -> ("error out"=w396:errorcluster, "Is Taps Supported"=w400:bool)  [unwired: 6 in, 1 out]
              n149 = case shown="False" w400 {
                tunnel: w399 -> [w405 w406]
                tunnel: [w403 w406] -> w398
                tunnel: w397 -> [w404 _]
                frame False {
                  n150 = Build Array (concatenate)(w405, w404) -> (w403:u32[])
                }
                frame True {
                }
              }
            }
            n151 = property on="DataRate" class="Enum (strict)"(error in=w390, "Disabled Items []"=w391) -> (error out=w381:errorcluster)  [unwired: 1 in, 1 out]
            n152 = property on="Taps" class="Enum (strict)"(error in=w385, "Disabled Items []"=w386) -> (error out=w380:errorcluster)  [unwired: 1 in, 1 out]
            n153 = Merge Errors(w381, w380) -> (w379:errorcluster)
          }
          event Value Change {
            n154 = event-data() -> ("NewVal"=w419:T2)  [unwired: 1 in, 5 out]
            n155 = call "Set Color Balance.vi"("error in (no error)"=w420, "NewVal"=w419, "Color Processor References"=w418, "TLCamera reference"=w421) -> ("error out"=w424:errorcluster, "TLCamera reference out"=w423:refnum<k24>)  [unwired: 6 in]
          }
          event "Start Camera": Value Change {
            w427 = T13."Disabled and Grayed Out" ("Disabled")
            n156 = event-data() -> ()  [unwired: 1 in, 6 out]
            n157 = property on="Start Camera" class="Bool (strict)"(error in=w426, "DisabledEnum"=w427, "Value"=FALSE ("Open Camera")) -> (error out=w425:errorcluster)  [unwired: 1 in, 1 out]
            n158 = property on="Binning" class="Clust (strict)"("DisabledEnum"=w427) -> ("Value"=w486:T4)  [unwired: 2 in, 2 out]
            n159 = property on="Region of Interest" class="Clust (strict)"("DisabledEnum"=w427) -> ("Value"=w485:T3)  [unwired: 2 in, 2 out]
            n160 = control-ref of="Frame Number"() -> (w469:refnum<vi>)
            n161 = control-ref of="Camera Image"() -> (w468:refnum<vi>)
            n162 = property on="Image Type" class="Enum (strict)"() -> ("Value"=w438:T7)  [unwired: 2 in, 2 out]
            n163 = property on="Data Rate" class="Clust (strict)"("DisabledEnum"=w427) -> ("Value"=w482:cluster{"DataRate":T5, "Taps":T6})  [unwired: 2 in, 2 out]
            n164 = call-poly "Set Parameters.vi"("error in (no error)"=w425, "Region of Interest"=w485, "Binning"=w486, "TLCamera reference in"=w472) -> ("error out"=w481:errorcluster, "TLCamera reference out"=w484:refnum<k24>)  [unwired: 6 in]
            n165 = property on="Frames per Trigger\n(zero for unlimited)" class="DigNum (strict)"() -> ("Value"=w483:u32)  [unwired: 2 in, 2 out]
            n166 = Unbundle By Name(w482) -> ("DataRate"=w431:T5, "Taps"=w444:T6)
            n167 = call-poly "Set Parameters.vi"("error in (no error)"=w481, "FramesPerTrigger_zeroForUnlimited"=w483, "TLCamera reference in"=w484) -> ("error out"=w435:errorcluster, "TLCamera reference out"=w434:refnum<k24>)  [unwired: 7 in]
            n168 = vi-ref "OnImageFrameAvailable Event Callback - TLCamera Main Color.vi"() -> ("vi reference"=w436:refnum<vi>)
            n169 = call "Get Is DataRate Supported.vi"("error in (no error)"=w435, "Data Rate"=w431, "TLCamera reference"=w434) -> ("error out"=w432:errorcluster, "Is DataRate Supported"=w430:bool, "TLCamera reference out"=w433:refnum<k24>)  [unwired: 6 in]
            n170 = case shown="True" w430 {
              tunnel: [w488 w494] -> w449
              tunnel: [w489 w493] -> w448
              tunnel: w433 -> [w489 w492]
              tunnel: w432 -> [w488 w491]
              tunnel: w431 -> [_ w490]
              frame False {
              }
              frame True {
                n171 = call-poly "Set Parameters.vi"("error in (no error)"=w491, "DataRate"=w490, "TLCamera reference in"=w492) -> ("error out"=w494:errorcluster, "TLCamera reference out"=w493:refnum<k24>)  [unwired: 7 in]
              }
            }
            n172 = call "Get Is Taps Supported.vi"("error in (no error)"=w449, "Taps"=w444, "TLCamera reference"=w448) -> ("error out"=w447:errorcluster, "Is Taps Supported"=w446:bool, "TLCamera reference out"=w445:refnum<k24>)  [unwired: 6 in]
            n173 = property on="Trigger Settings" class="Clust (strict)"("DisabledEnum"=w427) -> ("Value"=w480:T8)  [unwired: 2 in, 2 out]
            n174 = case shown="True" w446 {
              tunnel: [w496 w501] -> w440
              tunnel: [w495 w500] -> w439
              tunnel: w447 -> [w495 w498]
              tunnel: w445 -> [w496 w499]
              tunnel: w444 -> [_ w497]
              frame False {
              }
              frame True {
                n175 = call-poly "Set Parameters.vi"("error in (no error)"=w498, "Taps"=w497, "TLCamera reference in"=w499) -> ("error out"=w500:errorcluster, "TLCamera reference out"=w501:refnum<k24>)  [unwired: 7 in]
              }
            }
            n176 = call "Set Trigger Settings.vi"("error in (no error)"=w439, "Trigger Settings"=w480, "TLCamera reference"=w440) -> ("error out"=w465:errorcluster, "TLCamera reference out"=w464:refnum<k24>)  [unwired: 7 in]
            n177 = property on="Exposure (ms)" class="DigNum (strict)"() -> ("Value"=w443:dbl)  [unwired: 2 in, 2 out]
            n178 = Multiply(x=w443, y=1000.0) -> (x*y=w441:dbl)
            n179 = call-poly "Set Parameters.vi"("error in (no error)"=w465, "ExposureTime_us"=w441, "TLCamera reference in"=w464) -> ("error out"=w462:errorcluster, "TLCamera reference out"=w463:refnum<k24>)  [unwired: 7 in]
            n180 = property on="Black Level" class="DigNum (strict)"() -> ("Value"=w458:u32)  [unwired: 2 in, 2 out]
            n181 = call "Get Is BlackLevel Supported.vi"("error in (no error)"=w462, "TLCamera reference in"=w463) -> ("error out"=w459:errorcluster, "Is BlackLevel Supported?"=w461:bool, "TLCamera reference out"=w460:refnum<k24>)  [unwired: 7 in]
            n182 = case shown="True" w461 {
              tunnel: w460 -> [w510 w515]
              tunnel: w459 -> [w509 w514]
              tunnel: [w509 w513] -> w457
              tunnel: [w510 w512] -> w456
              tunnel: w458 -> [_ w511]
              frame False {
              }
              frame True {
                n183 = call-poly "Set Parameters.vi"("error in (no error)"=w514, "BlackLevel"=w511, "TLCamera reference in"=w515) -> ("error out"=w513:errorcluster, "TLCamera reference out"=w512:refnum<k24>)  [unwired: 7 in]
              }
            }
            n184 = property on="Image Type" class="Enum (strict)"("DisabledEnum"=w427) -> ()  [unwired: 2 in, 2 out]
            n185 = property on="Frame Settings" class="Clust (strict)"("DisabledEnum"=w427) -> ()  [unwired: 2 in, 2 out]
            n186 = Unbundle By Name(w480) -> ("Trigger Mode"=w479:T9)
            n187 = property on="Gain" class="DigNum (strict)"() -> ("Value"=w452:u32)  [unwired: 2 in, 2 out]
            n188 = call "Get Is Gain Supported.vi"("error in (no error)"=w457, "TLCamera reference in"=w456) -> ("error out"=w454:errorcluster, "Is Gain Supported?"=w453:bool, "TLCamera reference out"=w455:refnum<k24>)  [unwired: 7 in]
            n189 = case shown="True" w453 {
              tunnel: w455 -> [w503 w508]
              tunnel: w454 -> [w502 w507]
              tunnel: [w502 w506] -> w451
              tunnel: [w503 w505] -> w450
              tunnel: w452 -> [_ w504]
              frame False {
              }
              frame True {
                n190 = call-poly "Set Parameters.vi"("error in (no error)"=w507, "Gain"=w504, "TLCamera reference in"=w508) -> ("error out"=w506:errorcluster, "TLCamera reference out"=w505:refnum<k24>)  [unwired: 7 in]
              }
            }
            n191 = Bundle("TLCamera reference out"=w450, "Frame Number"=w469, "Camera Image"=w468, "Value"=w438, "Color Processor References"=w437) -> (w467:T14)  [unwired: 1 in]
            n192 = node(w451, w450, w436, w467) -> (→"event callback refnum":refnum<k27>, w470:errorcluster)  [unwired: 1 in]
            n193 = call "Arm TLCamera.vi"("error in (no error)"=w470, "TLCamera reference"=w450) -> ("error out"=w475:errorcluster, "TLCamera reference out"=w476:refnum<k24>)  [unwired: 8 in]
            n194 = Equal?(x=w479, y=Trigger_Modes."Software") -> (x = y?=w477:bool)
            n195 = case shown="True" w477 {
              tunnel: w476 -> [w517 w521]
              tunnel: w475 -> [w516 w520]
              tunnel: [w517 w519] -> w474
              tunnel: [w516 w518] -> w429
              frame False {
              }
              frame True {
                n196 = call "Issue Software Trigger.vi"("error in (no error)"=w520, "TLCamera Reference"=w521) -> ("error out"=w518:errorcluster, "TLCamera reference out"=w519:refnum<k24>)  [unwired: 8 in]
              }
            }
            n197 = property on="Stop Camera" class="Bool (strict)"(error in=w429, "DisabledEnum"=T13."Enabled" ("Disabled")) -> (error out=w471:errorcluster)  [unwired: 1 in, 1 out]
          }
          event "Stop Camera": Value Change {
            n198 = event-data() -> ("NewVal"=w523:bool)  [unwired: 1 in, 5 out]
            n199 = case shown="True" w523 {
              tunnel: w528 -> [w529 w548]
              tunnel: [w530 w538] -> w527
              tunnel: [w529 w537] -> w526
              tunnel: w524 -> [w530 w536]
              frame False {
              }
              frame True {
                w542 = T13."Enabled" ("Disabled")
                n200 = property on="event callback refnum" class="Ref (strict)"() -> ("Value"=w533:refnum<k27>)  [unwired: 2 in, 2 out]
                n201 = Not A Number/Path/Refnum?(number/path/refnum=w533) -> (NaN/Path/Refnum?=w535:bool)
                n202 = call "Disarm TLCamera.vi"("error in (no error)"=w548, "TLCamera reference"=w536) -> ("error out"=w534:errorcluster, "TLCamera reference out"=w538:refnum<k24>)  [unwired: 8 in]
                n203 = case shown="False" w535 {
                  tunnel: w534 -> [w550 w552]
                  tunnel: w533 -> [w551 _]
                  tunnel: [w549 w552] -> w532
                  frame False {
                    n204 = Unregister For Events(event registration refnum=w551, error in=w550) -> (error out=w549:errorcluster)
                  }
                  frame True {
                  }
                }
                n205 = property on="Data Rate" class="Clust (strict)"(error in=w532, "DisabledEnum"=w542) -> (error out=w547:errorcluster)  [unwired: 1 in, 1 out]
                n206 = property on="Frame Settings" class="Clust (strict)"(error in=w547, "DisabledEnum"=w542) -> (error out=w546:errorcluster)  [unwired: 1 in, 1 out]
                n207 = property on="Image Type" class="Enum (strict)"() -> ("Value"=w531:T7)  [unwired: 2 in, 2 out]
                n208 = property on="Image Type" class="Enum (strict)"(error in=w546, "DisabledEnum"=w542, "Val(Sgnl)"=w531) -> (error out=w545:errorcluster)  [unwired: 1 in, 1 out]
                n209 = property on="Region of Interest" class="Clust (strict)"(error in=w545, "DisabledEnum"=w542) -> (error out=w544:errorcluster)  [unwired: 1 in, 1 out]
                n210 = property on="Trigger Settings" class="Clust (strict)"(error in=w544, "DisabledEnum"=w542) -> (error out=w543:errorcluster)  [unwired: 1 in, 1 out]
                n211 = property on="Start Camera" class="Bool (strict)"(error in=w543, "DisabledEnum"=w542) -> (error out=w541:errorcluster)  [unwired: 1 in, 1 out]
                n212 = property on="Stop Camera" class="Bool (strict)"(error in=w541, "DisabledEnum"=T13."Disabled and Grayed Out" ("Disabled"), "Value"=FALSE ("Stop Camera")) -> (error out=w537:errorcluster)  [unwired: 1 in, 1 out]
              }
            }
          }
        }
        n213 = Unbundle By Name(w61) -> ("status"=w60:bool)
        n214 = case shown="False" w60 {
          tunnel: w59 -> [w68 _]
          tunnel: [w68 Status_-_Main."Close"] -> w58
          frame False {
          }
          frame True {
          }
        }
      }
      frame "Close" {
        w570 = T13."Disabled and Grayed Out" ("Disabled")
        n215 = call <vilib>:"Simple Error Handler.vi"("error in (no error)"=w562) -> ("error out"=w561:errorcluster)  [unwired: 4 in, 4 out]
        n216 = call <vilib>:"Clear Errors.vi"("error in (no error)"=w561) -> ("error out"=w560:errorcluster)  [unwired: 5 in, 1 out]
        n217 = property on="event callback refnum" class="Ref (strict)"(error in=w560) -> (error out=w564:errorcluster, "Value"=w565:refnum<k27>)  [unwired: 1 in, 1 out]
        n218 = Not A Number/Path/Refnum?(number/path/refnum=w565) -> (NaN/Path/Refnum?=w566:bool)
        n219 = case shown="False" w566 {
          tunnel: w565 -> [w584 _]
          tunnel: w564 -> [w583 w585]
          tunnel: [w582 w585] -> w563
          frame False {
            n220 = Unregister For Events(event registration refnum=w584, error in=w583) -> (error out=w582:errorcluster)
          }
          frame True {
          }
        }
        n221 = Not A Number/Path/Refnum?(number/path/refnum=w576) -> (NaN/Path/Refnum?=w577:bool)
        n222 = case shown="False" w577 {
          tunnel: w576 -> [w588 _]
          tunnel: w563 -> [w587 w589]
          tunnel: [w586 w589] -> w556
          frame False {
            n223 = call "Close TLCamera.vi"("error in (no error)"=w587, "TLCamera reference"=w588) -> ("error out"=w586:errorcluster)  [unwired: 9 in]
          }
          frame True {
          }
        }
        n224 = call "Close Color Processors.vi"("error in (no error)"=w556, "Color Processor References"=w554) -> ("error out"=w555:errorcluster)  [unwired: 9 in]
        n225 = call <vilib>:"Simple Error Handler.vi"("error in (no error)"=w555) -> ("error out"=w559:errorcluster)  [unwired: 4 in, 4 out]
        n226 = call <vilib>:"Clear Errors.vi"("error in (no error)"=w559) -> ("error out"=w558:errorcluster)  [unwired: 5 in, 1 out]
        n227 = call "Close TLCameraSDK.vi"("error in (no error)"=w558, "TLCameraSDK reference"=w581) -> ("error out"=w575:errorcluster)  [unwired: 9 in]
        n228 = property on="Start Camera" class="Bool (strict)"(error in=w575, "DisabledEnum"=w570) -> (error out=w574:errorcluster)  [unwired: 1 in, 1 out]
        n229 = property on="Stop Camera" class="Bool (strict)"(error in=w574, "DisabledEnum"=w570) -> (error out=w573:errorcluster)  [unwired: 1 in, 1 out]
        n230 = property on="Open Camera" class="Bool (strict)"(error in=w573, "DisabledEnum"=w570) -> (error out=w572:errorcluster)  [unwired: 1 in, 1 out]
        n231 = property on="Close Camera" class="Bool (strict)"(error in=w572, "DisabledEnum"=w570) -> (error out=w571:errorcluster)  [unwired: 1 in, 1 out]
        n232 = property on="Camera Settings" class="Clust (strict)"(error in=w571, "DisabledEnum"=w570) -> (error out=w569:errorcluster)  [unwired: 1 in, 1 out]
        n233 = property on="Refresh" class="Bool (strict)"(error in=w569, "DisabledEnum"=T13."Enabled" ("Disabled")) -> (error out=w568:errorcluster)  [unwired: 1 in, 1 out]
        n234 = property on="Exit" class="Bool (strict)"(error in=w568, "Value"=FALSE ("Exit")) -> (error out=w557:errorcluster)  [unwired: 1 in, 1 out]
      }
    }
    "Status" <- w6
  }
  n235 = call <vilib>:"Simple Error Handler.vi"("error in (no error)"=w1) -> ()  [unwired: 4 in, 5 out]
